vi "test_cpu-memory_usagwe.vi"() -> ()   [LabVIEW 2019]
panel:
  out "Mem. Usage":sgl format="%.7p"
  out "CPU Usage":sgl
  in  "정지":bool
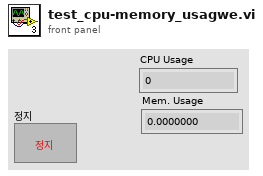
[diagram p1: front panel]
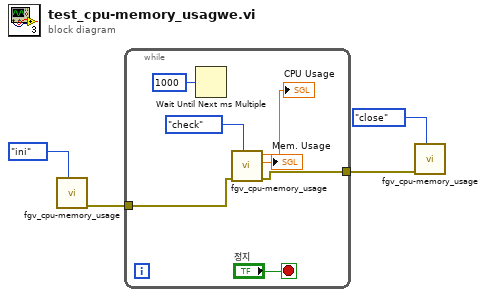
[diagram p0: block diagram]
diagram:
  n1 = call "fgv_cpu-memory_usage.vi"("cmd"=enum16{"ini", "check", "close"}."ini") -> ("error out"=w2:errorcluster)  [unwired: 8 in, 2 out]
  n2 = while {
    tunnel: w2 -> [w10]
    tunnel: [w8] -> w1
    stop <- "정지" stop-if-true
    n3 = Wait Until Next ms Multiple(millisecond multiple=u32 1000 ("대기 시간 (ms)")) -> ()  [unwired: 1 out]
    n4 = call "fgv_cpu-memory_usage.vi"("cmd"=enum16{"ini", "check", "close"}."check", "error in"=w10) -> ("error out"=w8:errorcluster, "Mem. Usage"=→"Mem. Usage":sgl, "CPU Usage"=→"CPU Usage":sgl)  [unwired: 7 in]
  }
  n5 = call "fgv_cpu-memory_usage.vi"("cmd"=enum16{"ini", "check", "close"}."close", "error in"=w1) -> ()  [unwired: 7 in, 3 out]
